vi "Measurement UI.vi"() -> ()   [LabVIEW 2021, in "Noise Sweep_Class D Amplifier_UI.lvlib"]
uses:
  Noise Sweep_Class D Amplifier_UI.lvlib
  shared/ui/controls/view.ctl
  shared/DAQmx/input terminal configuration.ctl
  UI State.ctl
  <vilib>/Utility/miscctls.llb/LVBoundsTypeDef.ctl
  <vilib>/Utility/miscctls.llb/LVPoint32TypeDef.ctl
  <vilib>/Utility/miscctls.llb/LVPointTypeDef.ctl
  shared/ui/UI Helpers.lvlib
  shared/audio popup ui/Audio Popup UI.lvlib
  shared/DAQmx/DAQmx utility.lvlib
panel:
  in  "view legend":T1
  out "plot point":string
  out "Sweep graph":cluster{"frequency (Hz)":dbl[], "THD+N":dbl[]}[](graph)
  out "Time domain graph":waveform(dbl)[](graph)
  out "channel names":string[](array[string])
  in  "digital serial cfg file":string
  in  "power supply resource":string="PXI1Slot4/ai0"
  out "idle channel noise (Vrms)":dbl[](array[numeric])
  out "power supply voltage (V)":dbl[](array[numeric])
  in  "Configuration tab":enum32{"Protocol", "Measurement"}(tab)
  out "digital serial file name":string
  in  "configure digital serial":bool
  in  "master clock channel list":string caption="Master Clock Channel"
  in  "digital channel list":string caption="Digital Audio Channel"
  in  "delay before measurement (s)":dbl=0.1 caption="Delay before measurement" format="%#_6ps"
  in  "input terminal cfg":T2 caption="Terminal Configuration"
  in  "input range":dbl=0.1 caption="Input range" format="%#_6g V"
  in  "power supply current limit":dbl caption="Current Limit" format="%#_g A"
  in  "power supply resource":refnum<k15> caption="Resource"
  in  "sweep number of steps":u32=20000 caption="Number of steps"
  in  "power supply voltage start":dbl=20.0 caption="Sweep start" format="%#_6p V"
  in  "power supply voltage stop":dbl=20000.0 caption="Sweep stop" format="%#_6g V"
  in  "Acquisition channel":tag
  in  "acq sampling rate":dbl=51200.0 caption="Sample rate" format="%#.6pHz"
  in  "measurement time (s)":dbl=0.1 caption="Minimum measurement time" format="%#_6ps"
  in  "weighting filter":T3(ring)=enum."A-weighting" caption="Weighting filter"
  out "wfm - data":dbl[](array[numeric])
  out "wfm - dt":dbl
  in  "acq channel":string="PXI1Slot4/ai0"
  # "hidden controls - used to sync with MeasLink"
  # "hidden indicators"
  # "Digital Serial Settings"
  # "Harware Resource"
  # "Power Supply Sweep"
  # "Filters"
  # "Acquisition"
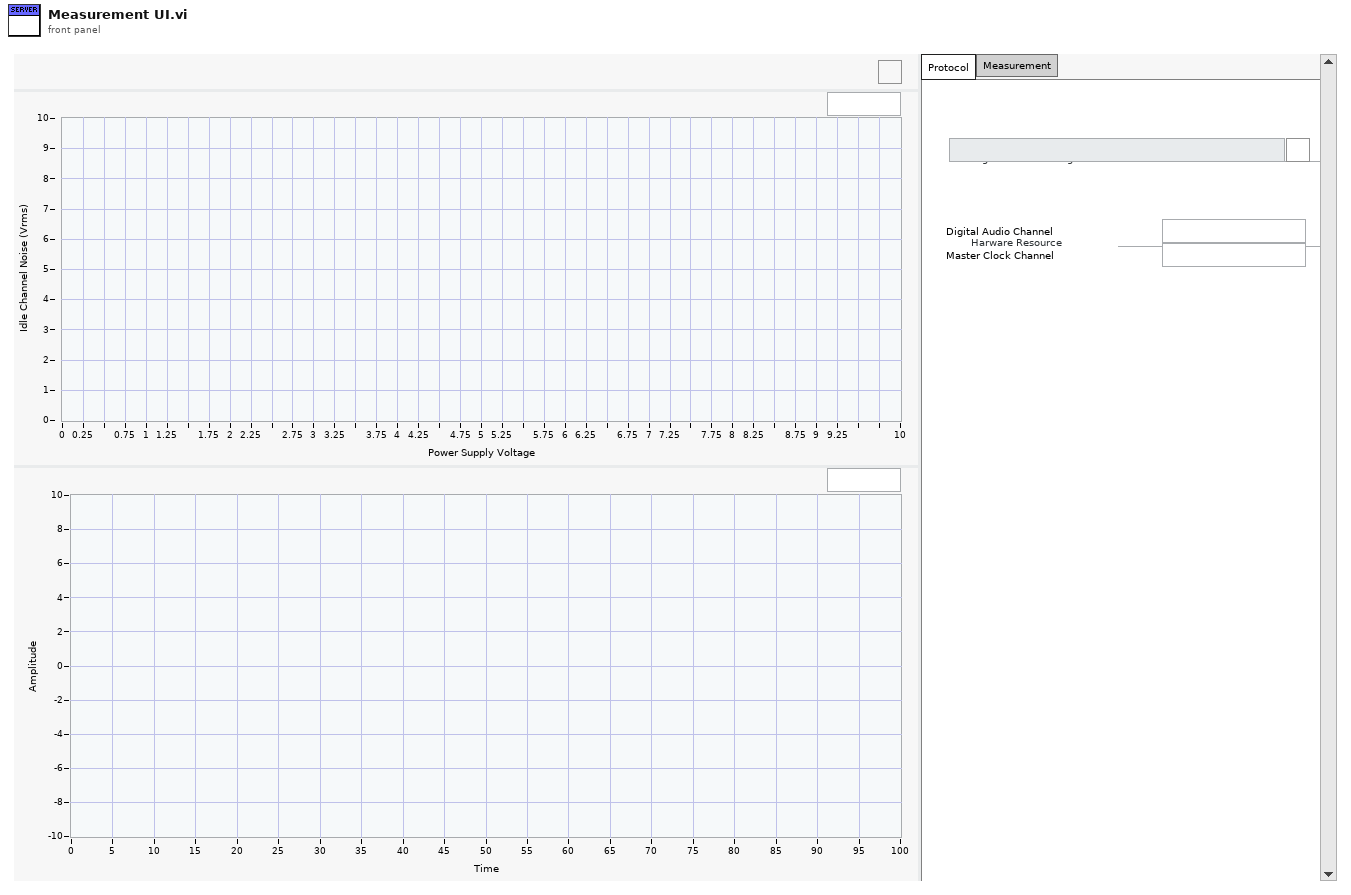
[diagram p1: front panel]
types:
  T1 = typedef "UI Helpers.lvlib/view.ctl" = bool
  T2 = typedef "DAQmx utility.lvlib/input terminal configuration.ctl" = enum32{"Default", "NRSE", "RSE", "Differential", "Pseudodifferential"}
  T3 = enum32{"Linear", "A-weighting", "B-weighting", "C-weighting"}
  T4 = typedef "Noise Sweep_Class D Amplifier_UI.lvlib/UI State.ctl" = cluster{"Graph Size":T5, "Legend Visible":bool, "Mouse Coords":T6, "Visible Plot Id":i32, "PostUI event occurred":bool, "digital serial cfg file":path}
  T5 = typedef "LVBoundsTypeDef.ctl" = cluster{"Width":u32, "Height":u32}
  T6 = typedef "LVPoint32TypeDef.ctl" = cluster{"Horizontal":i32, "Vertical":i32}
  T7 = typedef "LVPointTypeDef.ctl" = cluster{"Horizontal":i16, "Vertical":i16}
  T8 = typedef "Audio Popup UI.lvlib/audio settings.ctl" = cluster{"digital serial file":string}
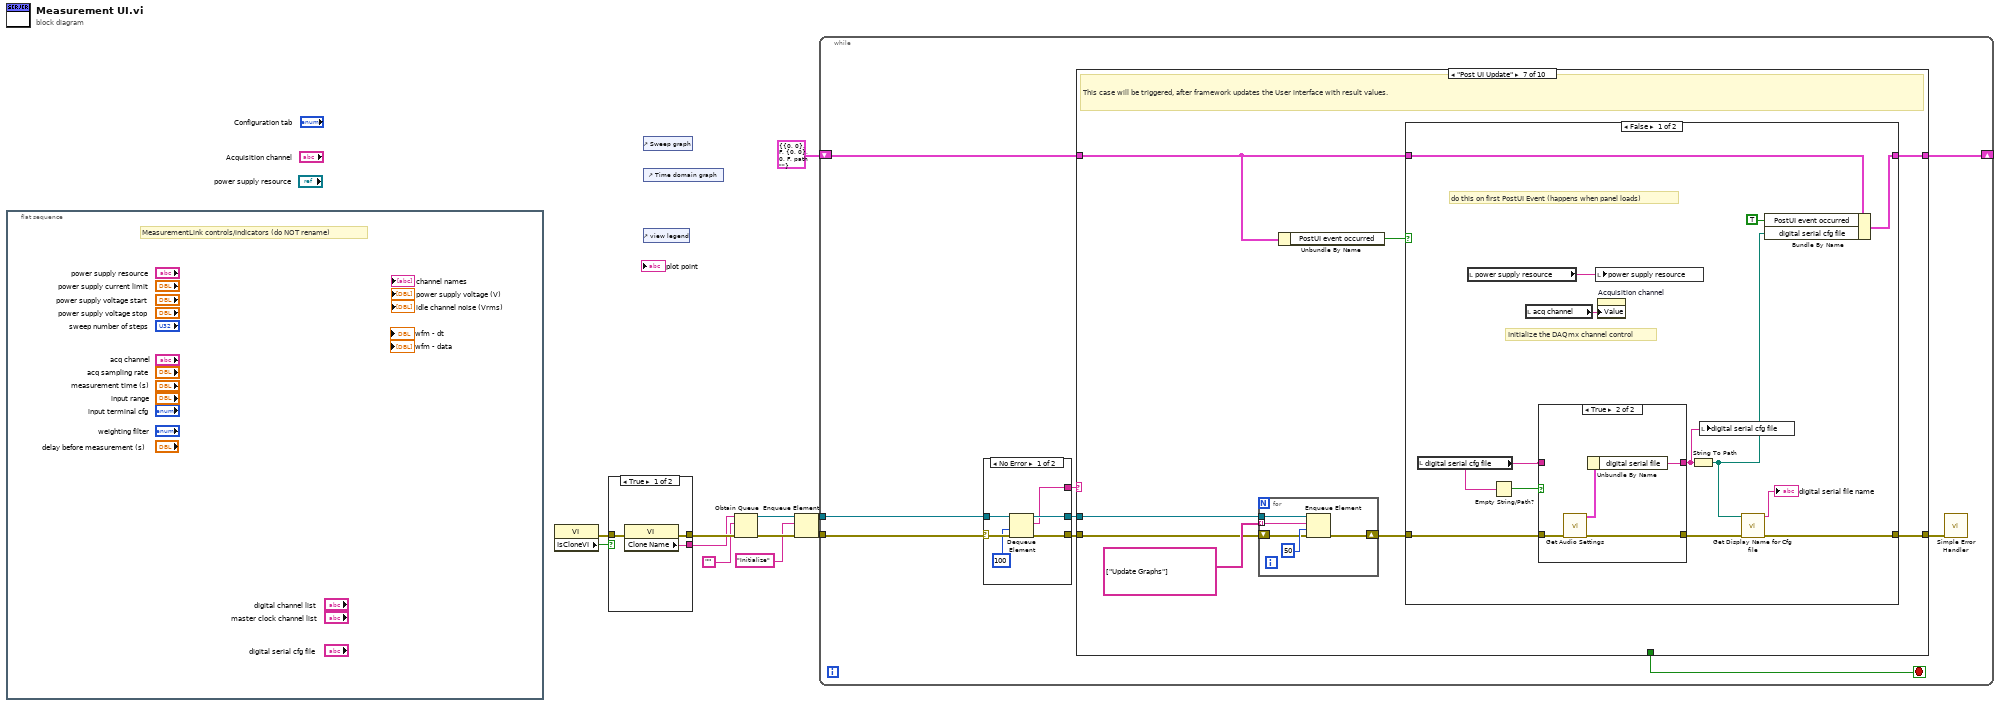
[diagram p0: block diagram]
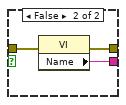
[diagram p2: hidden frame]
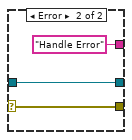
[diagram p3: hidden frame]
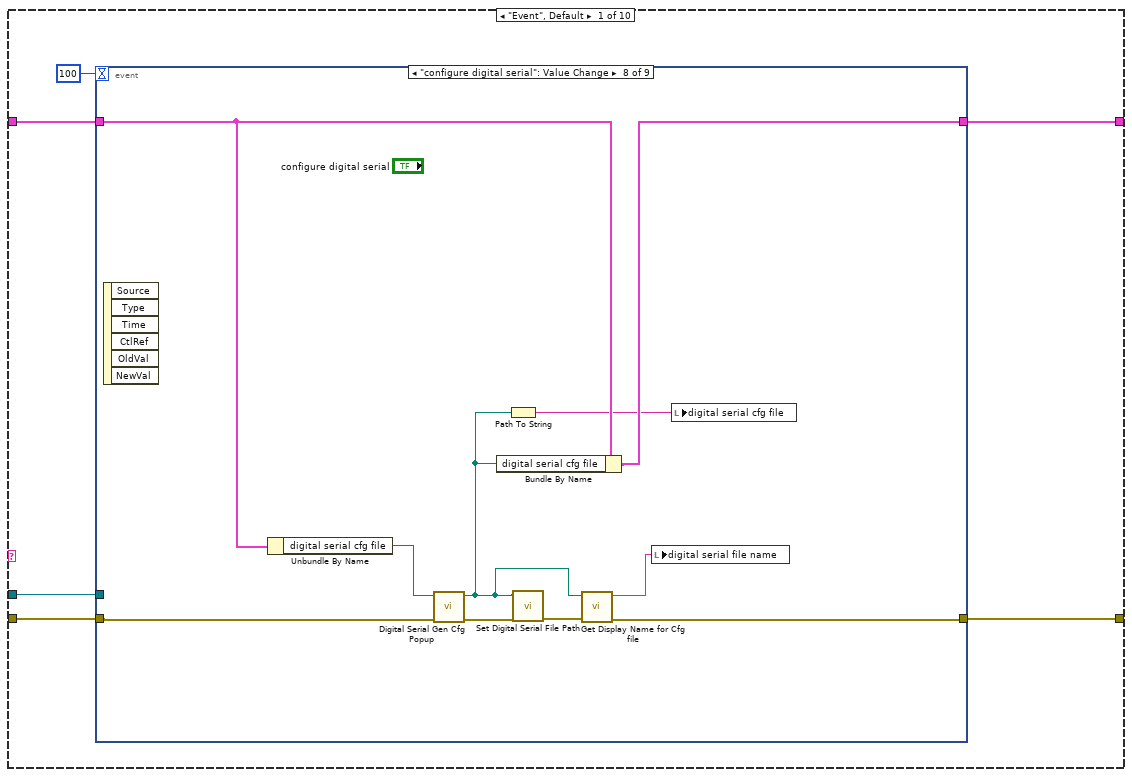
[diagram p4: hidden frame]
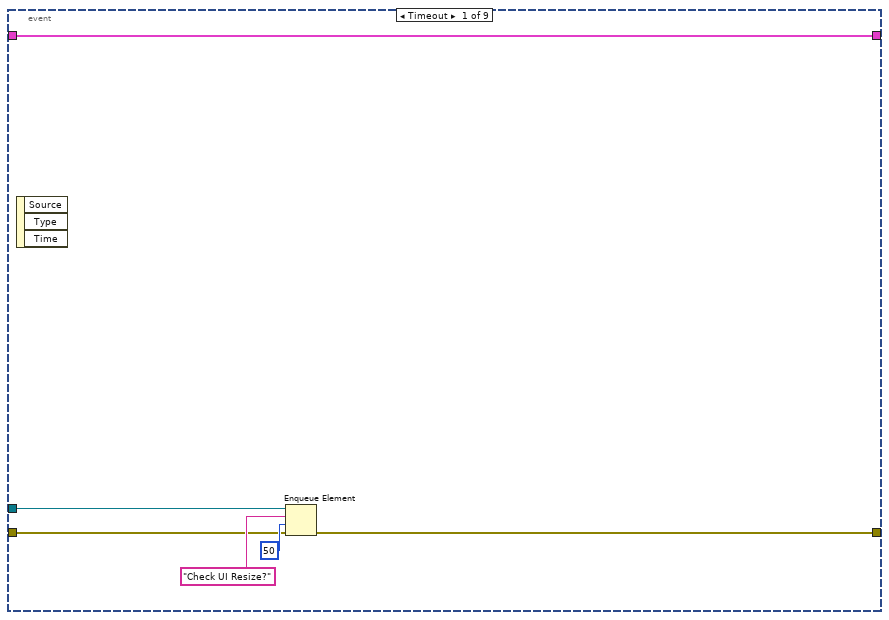
[diagram p5: hidden frame]
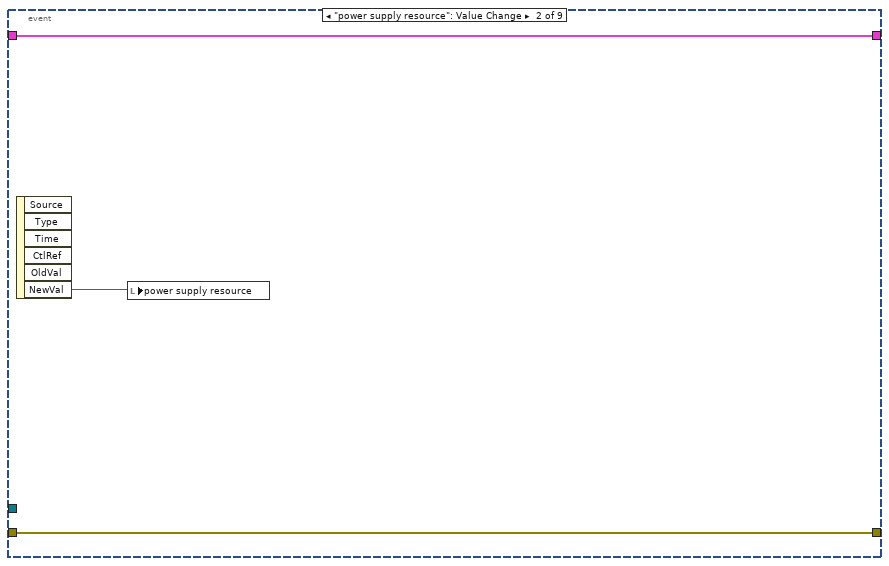
[diagram p6: hidden frame]
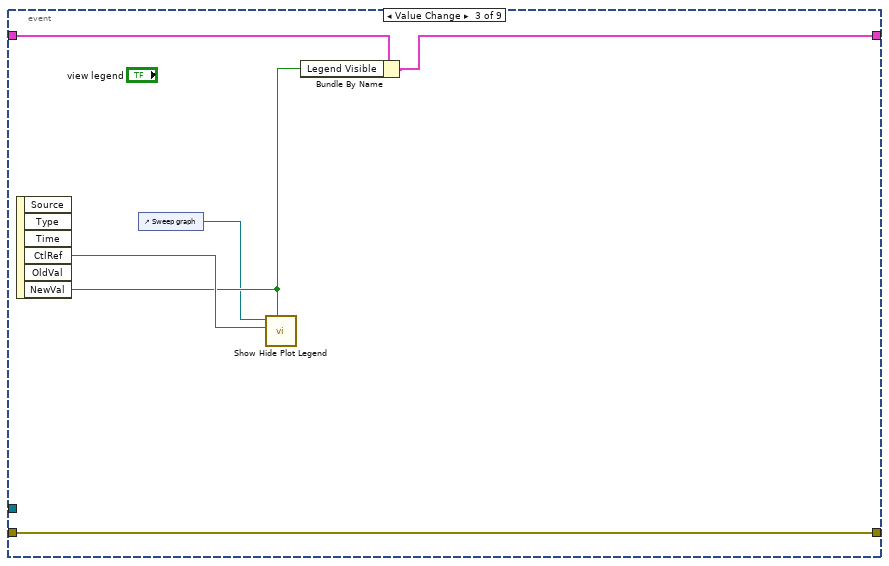
[diagram p7: hidden frame]
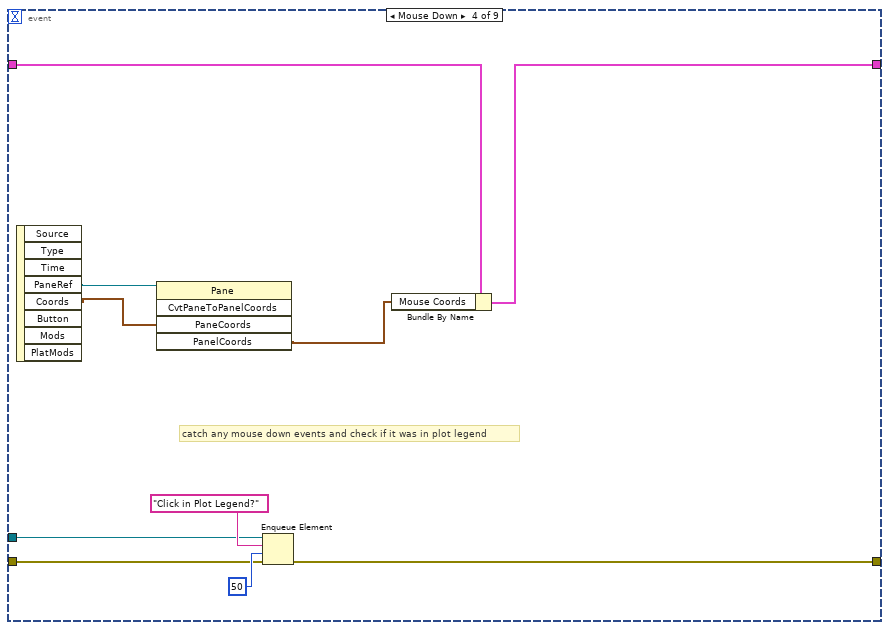
[diagram p8: hidden frame]
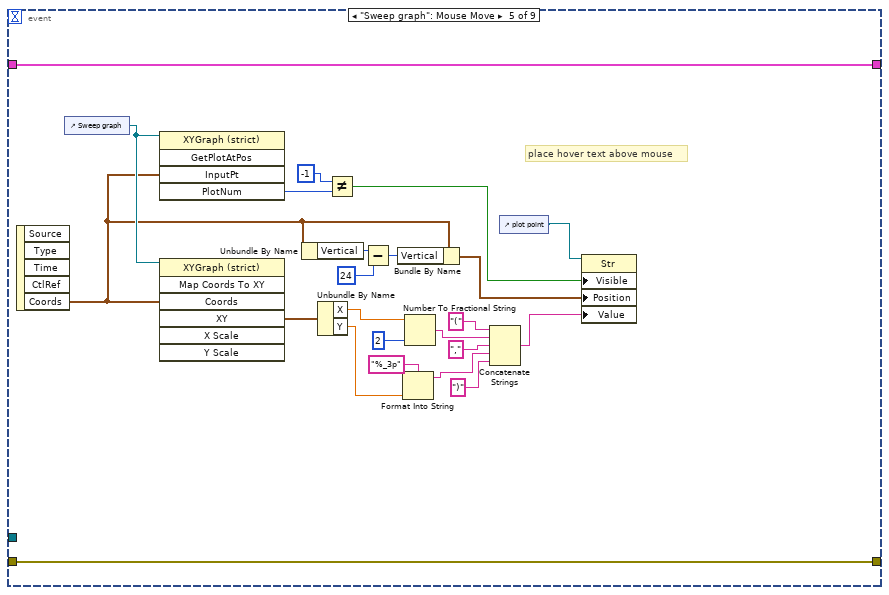
[diagram p9: hidden frame]
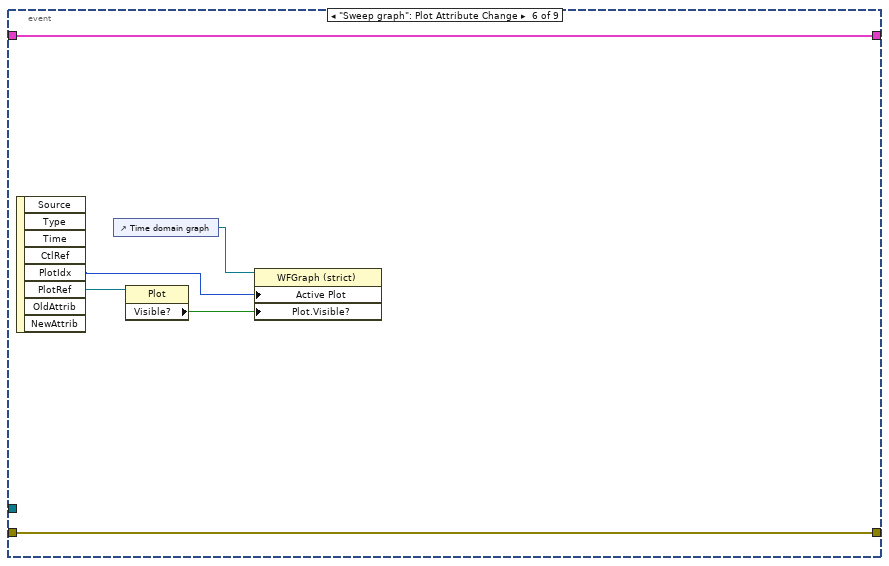
[diagram p10: hidden frame]
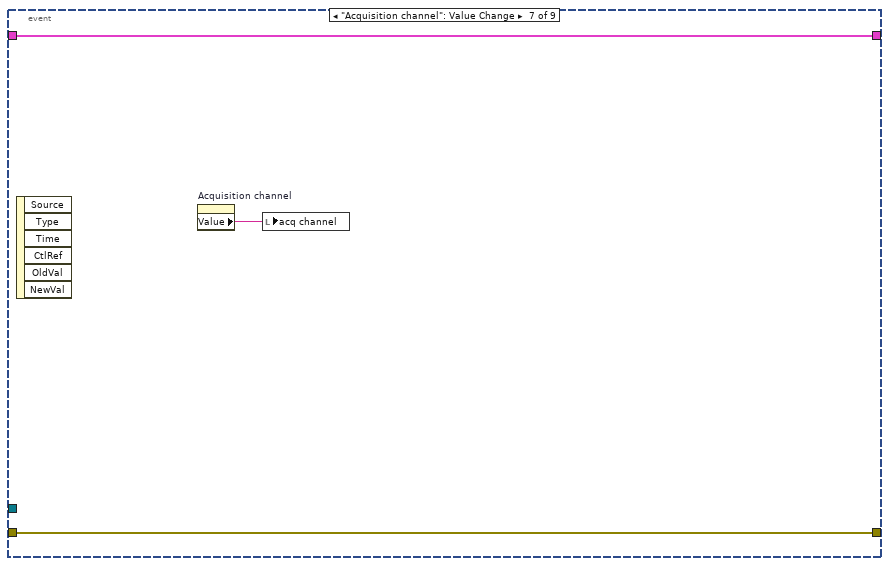
[diagram p11: hidden frame]
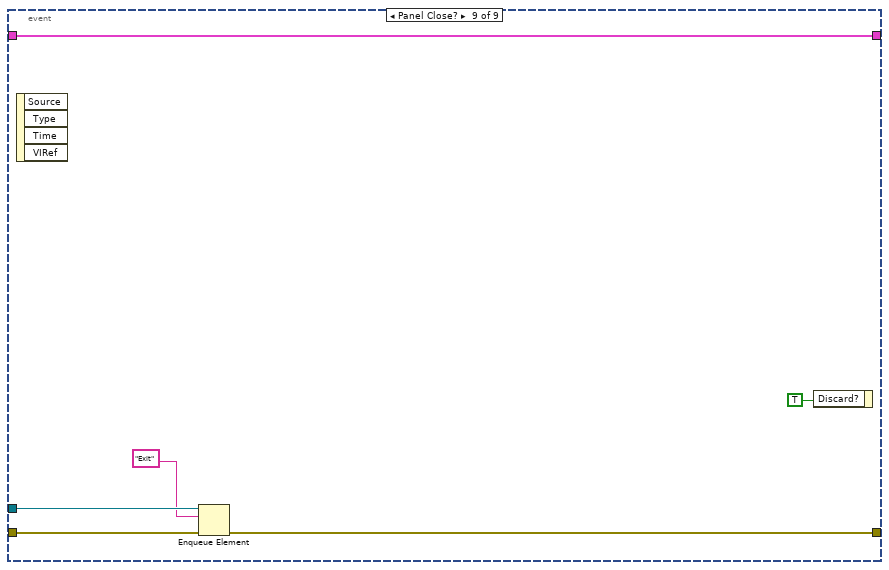
[diagram p12: hidden frame]
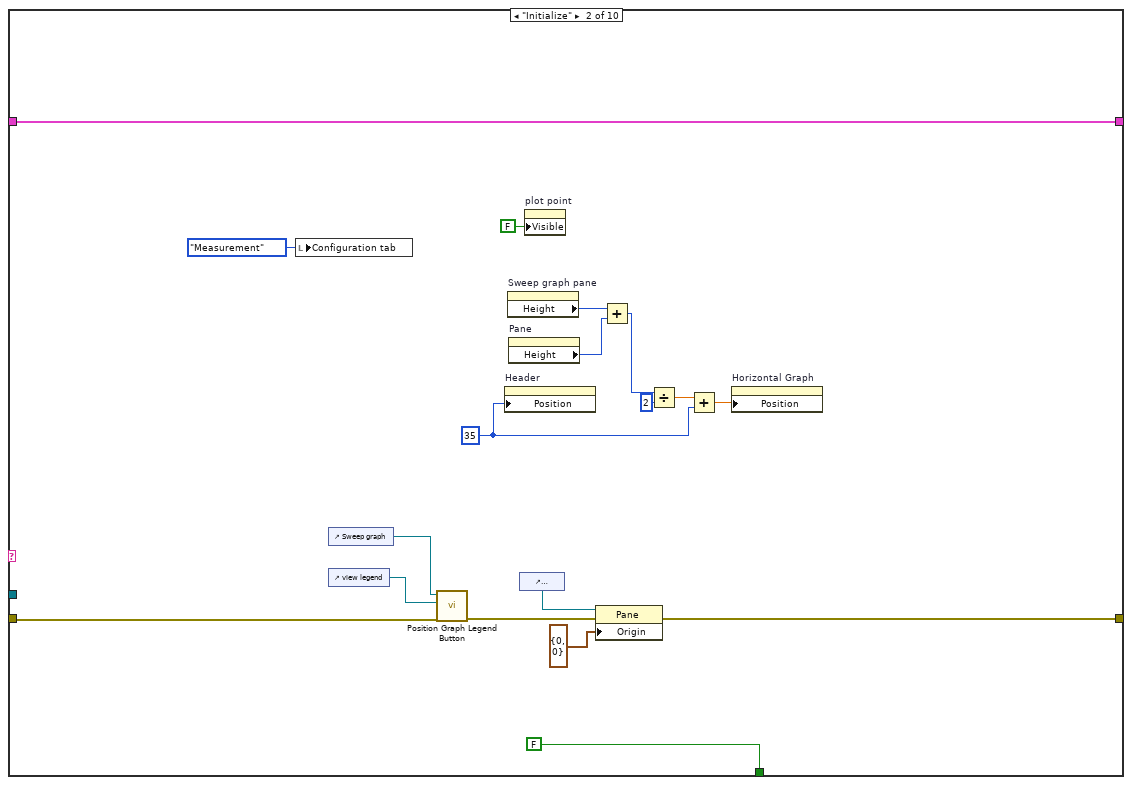
[diagram p13: hidden frame]
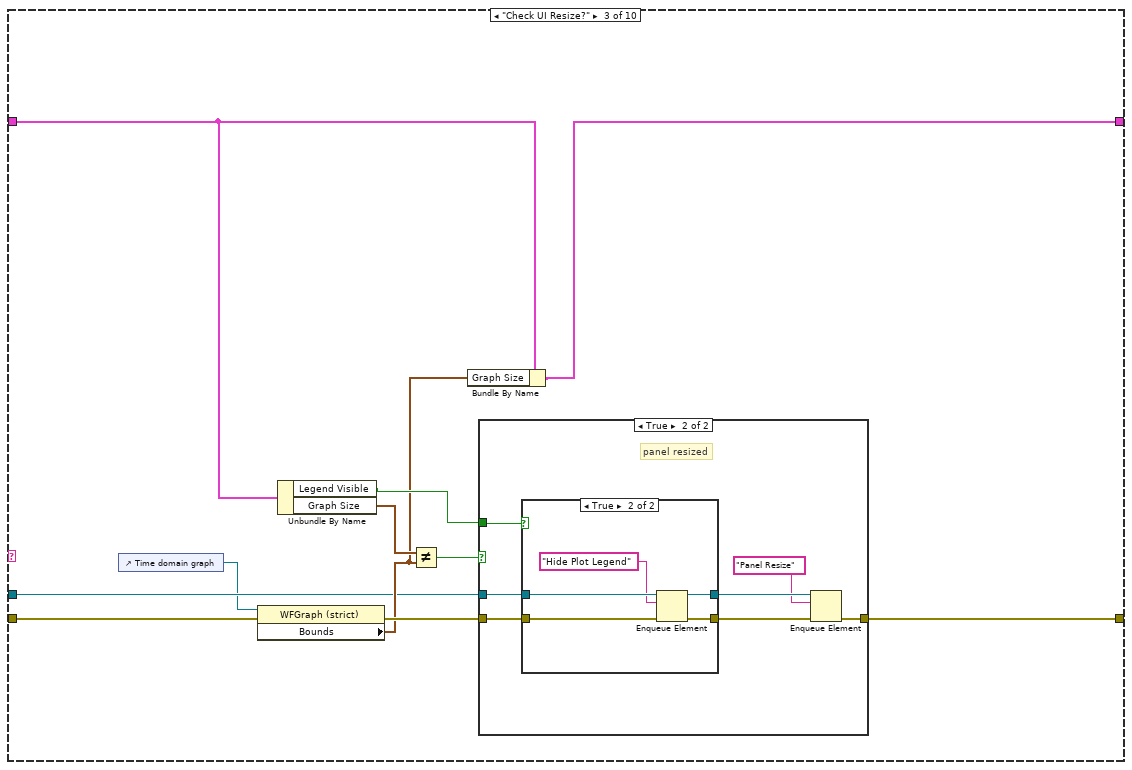
[diagram p14: hidden frame]
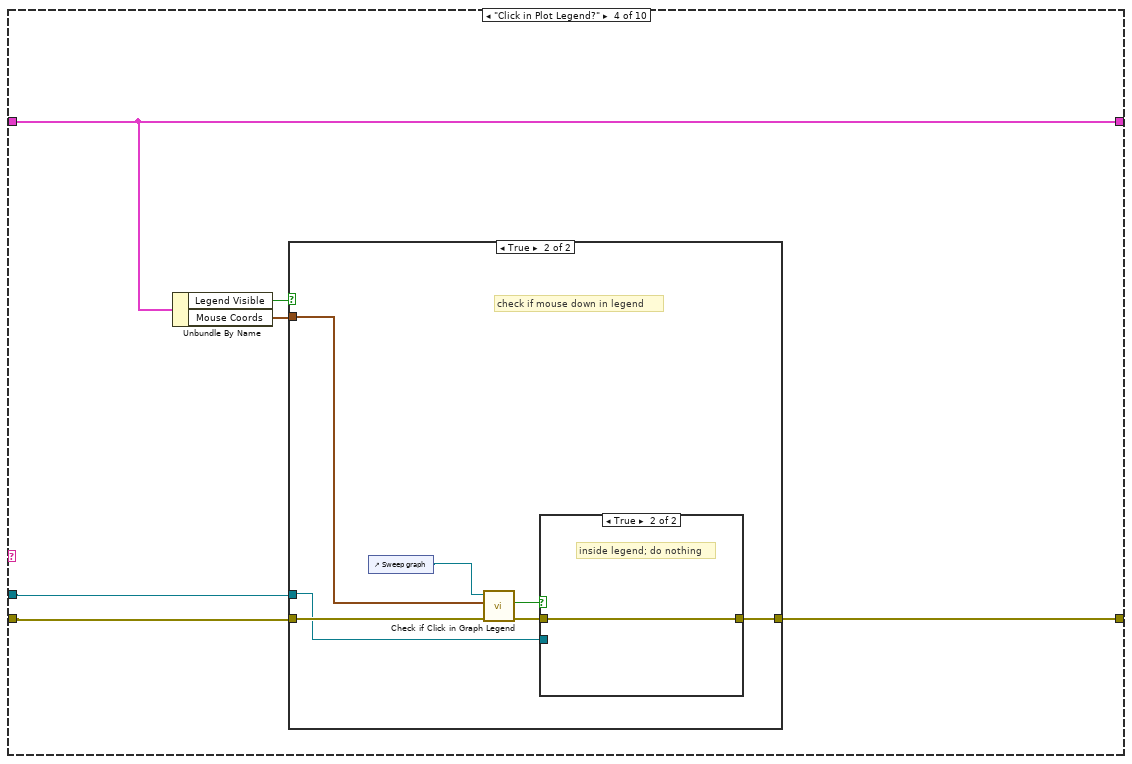
[diagram p17: hidden frame]
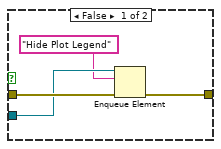
[diagram p19: hidden frame]
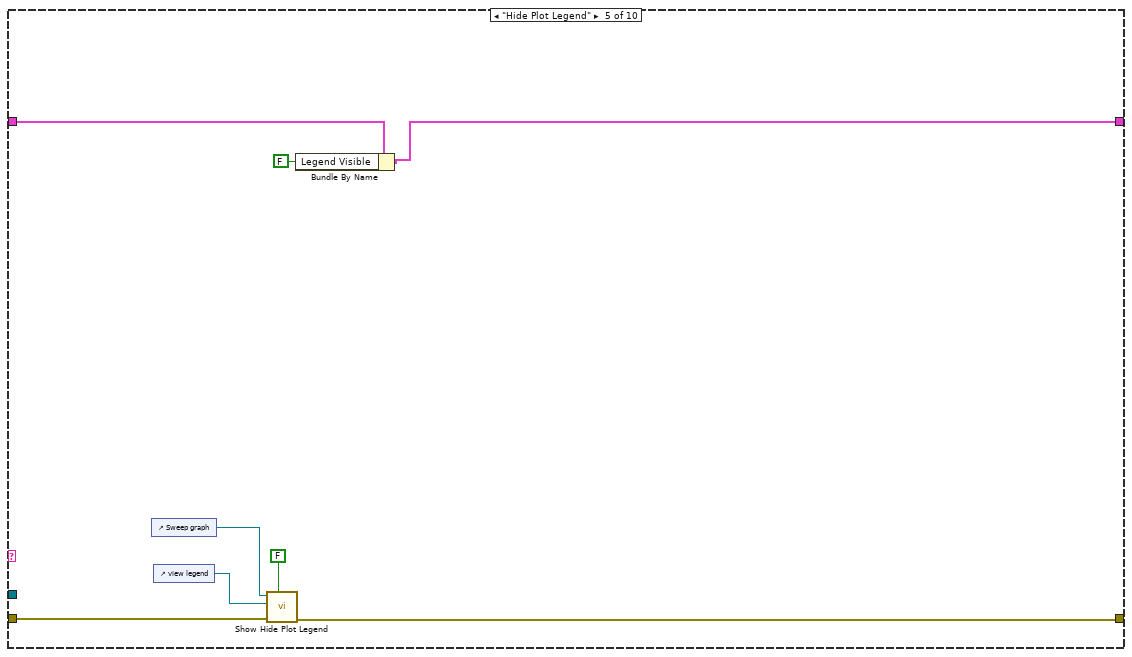
[diagram p20: hidden frame]
diagram:
  n1 = flat-sequence {
    frame #0 {
      # "MeasurementLink controls/indicators (do NOT rename)"
    }
  }
  n2 = property class="VI"() -> (error out=w2:errorcluster, "IsCloneVI"=w3:bool)  [unwired: 2 in, 1 out]
  n3 = case shown="True" w3 {
    tunnel: [w14 w17] -> w11
    tunnel: [w13 w16] -> w10
    tunnel: w2 -> [w12 w15]
    frame True {
      n4 = property class="VI"(error in=w12) -> (error out=w14:errorcluster, "Clone Name"=w13:string)  [unwired: 1 in, 1 out]
    }
    frame False {
      n5 = property class="VI"(error in=w15) -> (error out=w17:errorcluster, "Name"=w16:string)  [unwired: 1 in, 1 out]
    }
  }
  n6 = control-ref of="Sweep graph"() -> ()  [unwired: 1 out]
  n7 = control-ref of="Time domain graph"() -> ()  [unwired: 1 out]
  n8 = control-ref of="view legend"() -> ()  [unwired: 1 out]
  n9 = Obtain Queue(name (unnamed)=w10, element data type="", error in (no error)=w11) -> (queue out=w7:refnum<queue>, error out=w9:errorcluster)  [unwired: 2 in, 1 out]
  n10 = Enqueue Element(queue=w7, element="Initialize", error in (no error)=w9) -> (queue out=w6:refnum<queue>, error out=w8:errorcluster)  [unwired: 1 in, 1 out]
  n11 = while {
    tunnel: w6 -> [w24]
    shift-right: [w20] -> _
    shift-left: T4 {"Graph Size"={"Width"=0, "Height"=0}, "Legend Visible"=FALSE, "Mouse Coords"={"Horizontal"=0, "Vertical"=0}, "Visible Plot Id"=0, "PostUI event occurred"=FALSE, "digital serial cfg file"=path ""} ("UI State") -> [w19]
    tunnel: w8 -> [w26]
    stop <- w21 stop-if-true
    n12 = case shown="No Error" w26 {
      selector: w26 -> [w32 w35]
      tunnel: [w31 w35] -> w25
      tunnel: w24 -> [w30 w34]
      tunnel: [w29 w34] -> w23
      tunnel: [w28 "Handle Error"] -> w22
      frame No Error {
        n13 = Dequeue Element(queue=w30, timeout in ms (-1)=100, error in (no error)=w32) -> (queue out=w29:refnum<queue>, element=w28:string, error out=w31:errorcluster)  [unwired: 1 out]
      }
      frame Error {
      }
    }
    n14 = case shown="\"Post UI Update\"" w22 {
      tunnel: w25 -> [w40 w116 w137 w161 w181 w189 w197 w237 w253 w255]
      tunnel: w23 -> [w38 _ w138 w162 _ _ w196 _ w251 _]
      tunnel: [w41 w117 w136 w160 w180 w188 w191 w237 w248 w255] -> w18
      tunnel: [_ FALSE _ _ _ _ _ _ TRUE _] -> w21
      tunnel: [w36 w122 w133 w159 w183 w190 w194 w236 w246 w254] -> w20
      tunnel: w19 -> [w37 w122 w134 w159 w184 w190 w195 w236 w246 w254]
      frame "Event", Default {
        n15 = event shown="[7] \"configure digital serial\": Value Change" {
          selector: _ -> [_ _ _ _ _ _ _ _ _]
          dyn-events: _ -> [_ _ _ _ _ _ _ _ _]
          timeout: 100 -> [_ _ _ _ _ _ _ _ _]
          tunnel: [w44 w50 w56 w62 w89 w94 w96 w99 w112] -> w41
          tunnel: w40 -> [w45 w50 w56 w64 w89 w94 w96 w104 w113]
          tunnel: w38 -> [w43 _ _ w63 _ _ _ _ w111]
          tunnel: w37 -> [w42 w49 w53 w61 w88 w93 w97 w103 w109]
          tunnel: [w42 w49 w52 w60 w88 w93 w97 w102 w109] -> w36
          event Timeout {
            n16 = event-data() -> ()  [unwired: 1 in, 3 out]
            n17 = Enqueue Element(queue=w43, element="Check UI Resize?", timeout in ms (-1)=50, error in (no error)=w45) -> (error out=w44:errorcluster)  [unwired: 2 out]
          }
          event "power supply resource": Value Change {
            n18 = event-data() -> ("NewVal"=w48:refnum<k15>)  [unwired: 1 in, 5 out]
            n19 = local write "power supply resource"(w48) -> ()
          }
          event Value Change {
            n20 = event-data() -> ("CtlRef"=w55:refnum<vi>, "NewVal"=w54:T1)  [unwired: 1 in, 4 out]
            n21 = control-ref of="Sweep graph"() -> (w51:refnum<vi>)
            n22 = call "Show Hide Plot Legend.vi"("show"=w54, "view reference"=w55, "graph reference"=w51) -> ()  [unwired: 8 in, 1 out]
            n23 = Bundle By Name(cluster=w53, "Legend Visible"=w54) -> (w52:T4)
          }
          event Mouse Down {
            # "catch any mouse down events and check if it was in plot legend"
            n24 = event-data() -> ("PaneRef"=w59:refnum<vi>, "Coords"=w58:T6)  [unwired: 1 in, 6 out]
            n25 = invoke class="Pane" method="CvtPaneToPanelCoords"(reference=w59, "PaneCoords"=w58) -> ("PanelCoords"=w57:T7)  [unwired: 3 in, 4 out]
            n26 = Enqueue Element(queue=w63, element="Click in Plot Legend?", timeout in ms (-1)=50, error in (no error)=w64) -> (error out=w62:errorcluster)  [unwired: 2 out]
            n27 = Bundle By Name(cluster=w61, "Mouse Coords"=w57) -> (w60:T4)
          }
          event "Sweep graph": Mouse Move {
            # "place hover text above mouse"
            n28 = event-data() -> ("Coords"=w70:T6)  [unwired: 1 in, 4 out]
            n29 = control-ref of="Sweep graph"() -> (w71:refnum<vi>)
            n30 = invoke class="XYGraph (strict)" method="GetPlotAtPos"(reference=w71, "InputPt"=w70) -> ("PlotNum"=w86:i32)  [unwired: 3 in, 4 out]
            n31 = invoke class="XYGraph (strict)" method="Map Coords To XY"(reference=w71, "Coords"=w70) -> ("XY"=w87:cluster{"X":dbl, "Y":dbl})  [unwired: 5 in, 6 out]
            n32 = Unbundle By Name(w70) -> ("Vertical"=w75:i32)
            n33 = Unbundle By Name(w87) -> ("X"=w77:dbl, "Y"=w69:dbl)
            n34 = Not Equal?(x=-1, y=w86) -> (x != y?=w84:bool)
            n35 = Subtract(x=w75, y=24) -> (x-y=w74:i32)
            n36 = Bundle By Name(cluster=w70, "Vertical"=w74) -> (w76:T6)
            n37 = Format Into String(format string="%_3p", w69) -> (resulting string=w68:string)  [unwired: 2 in, 1 out]
            n38 = Number To Fractional String(number=w77, precision (6)=i16 2) -> (F-format string=w82:string)  [unwired: 2 in]
            n39 = Concatenate Strings("(" ("string"), w82, "," ("string"), w68, ")" ("string")) -> (w78:string)
            n40 = control-ref of="plot point"() -> (w72:refnum<vi>)
            n41 = property on="Property Node" class="Str"(reference=w72, "Visible"=w84, "Position"=w76, "Value"=w78) -> ()  [unwired: 1 in, 2 out]
          }
          event "Sweep graph": Plot Attribute Change {
            n42 = event-data() -> ("PlotIdx"=w92:i32, "PlotRef"=w95:refnum<vi>)  [unwired: 1 in, 6 out]
            n43 = control-ref of="Time domain graph"() -> (w90:refnum<vi>)
            n44 = property class="Plot"(reference=w95) -> ("Visible?"=w91:bool)  [unwired: 1 in, 2 out]
            n45 = property on="Property Node" class="WFGraph (strict)"(reference=w90, "Active Plot"=w92, "Plot.Visible?"=w91) -> ()  [unwired: 1 in, 2 out]
          }
          event "Acquisition channel": Value Change {
            n46 = event-data() -> ()  [unwired: 1 in, 6 out]
            n47 = property on="Acquisition channel" class="DAQmxName"() -> ("Value"=w98:string)  [unwired: 2 in, 2 out]
            n48 = local write "acq channel"(w98) -> ()
          }
          event "configure digital serial": Value Change {
            n49 = event-data() -> ()  [unwired: 1 in, 6 out]
            n50 = Unbundle By Name(w103) -> ("digital serial cfg file"=w108:path)
            n51 = call "Digital Serial Gen Cfg Popup.vi"("error in (no error)"=w104, "config file in"=w108) -> ("error out"=w107:errorcluster, "config file out"=w105:path)  [unwired: 7 in, 1 out]
            n52 = Bundle By Name(cluster=w103, "digital serial cfg file"=w105) -> (w102:T4)
            n53 = Path To String(path=w105) -> (string=w101:string)
            n54 = call "Set Digital Serial File Path.vi"("error in (no error)"=w107, "digital serial file"=w105) -> ("error out"=w106:errorcluster)  [unwired: 9 in]
            n55 = call "Get Display Name for Cfg file.vi"("error in (no error)"=w106, "file path"=w105) -> ("error out"=w99:errorcluster, "display string"=w100:string)  [unwired: 8 in]
            n56 = local write "digital serial file name"(w100) -> ()
            n57 = local write "digital serial cfg file"(w101) -> ()
          }
          event Panel Close? {
            n58 = event-data() -> ()  [unwired: 1 in, 4 out]
            n59 = Enqueue Element(queue=w111, element="Exit", error in (no error)=w113) -> (error out=w112:errorcluster)  [unwired: 1 in, 2 out]
            n60 = event-data("Discard?"=TRUE) -> ()  [unwired: 1 in, 1 out]
          }
        }
      }
      frame "Initialize" {
        w126 = 35 ("Splitter Position")
        n61 = local write "Configuration tab"(enum32{"Protocol", "Measurement"}."Measurement" ("Configuration tab")) -> ()
        n62 = control-ref of="Sweep graph"() -> (w127:refnum<vi>)
        n63 = control-ref of="view legend"() -> (w131:refnum<vi>)
        n64 = call "Position Graph Legend Button.vi"("error in (no error)"=w116, "view legend"=w131, "graph"=w127) -> ("error out"=w118:errorcluster)  [unwired: 8 in]
        n65 = property on="Header" class="Splitter"("Position"=w126) -> ()  [unwired: 2 in, 2 out]
        n66 = property on="Sweep graph pane" class="Pane"() -> ("Height"=w120:u32)  [unwired: 2 in, 2 out]
        n67 = property on="Pane" class="Pane"() -> ("Height"=w119:u32)  [unwired: 2 in, 2 out]
        n68 = control-ref of="Configuration Pane"() -> (w125:refnum<vi>)
        n69 = property on="plot point" class="Str"("Visible"=FALSE) -> ()  [unwired: 2 in, 2 out]
        n70 = property class="Pane"(reference=w125, error in=w118, "Origin"=T7 {"Horizontal"=0, "Vertical"=0}) -> (error out=w117:errorcluster)  [unwired: 1 out]
        n71 = Add(x=w120, y=w119) -> (x+y=w121:u32)
        n72 = Divide(x=w121, y=2) -> (x/y=w129:dbl)
        n73 = Add(x=w129, y=w126) -> (x+y=w128:dbl)
        n74 = property on="Horizontal Graph" class="Splitter"("Position"=w128) -> ()  [unwired: 2 in, 2 out]
      }
      frame "Check UI Resize?" {
        n75 = control-ref of="Time domain graph"() -> (w135:refnum<vi>)
        n76 = property on="Property Node" class="WFGraph (strict)"(reference=w135, error in=w137) -> (error out=w143:errorcluster, "Bounds"=w139:T5)  [unwired: 1 out]
        n77 = Unbundle By Name(w134) -> ("Legend Visible"=w141:bool, "Graph Size"=w140:T5)
        n78 = Not Equal?(x=w140, y=w139) -> (x != y?=w142:bool)
        n79 = Bundle By Name(cluster=w134, "Graph Size"=w139) -> (w133:T4)
        n80 = case shown="True" w142 {
          tunnel: w143 -> [w144 w151]
          tunnel: [w144 w146] -> w136
          tunnel: w141 -> [_ w149]
          tunnel: w138 -> [_ w150]
          frame False {
            # "no resize"
          }
          frame True {
            # "panel resized"
            n81 = case shown="True" w149 {
              tunnel: w151 -> [w153 w158]
              tunnel: [w153 w157] -> w148
              tunnel: w150 -> [w152 w156]
              tunnel: [w152 w154] -> w147
              frame False {
              }
              frame True {
                n82 = Enqueue Element(queue=w156, element="Hide Plot Legend", error in (no error)=w158) -> (queue out=w154:refnum<queue>, error out=w157:errorcluster)  [unwired: 1 in, 1 out]
              }
            }
            n83 = Enqueue Element(queue=w147, element="Panel Resize", error in (no error)=w148) -> (error out=w146:errorcluster)  [unwired: 1 in, 2 out]
          }
        }
      }
      frame "Click in Plot Legend?" {
        n84 = Unbundle By Name(w159) -> ("Legend Visible"=w163:bool, "Mouse Coords"=w164:T6)
        n85 = case shown="True" w163 {
          tunnel: w164 -> [_ w171]
          tunnel: w162 -> [_ w168]
          tunnel: w161 -> [w165 w172]
          tunnel: [w165 w167] -> w160
          frame False {
            # "legend not visible; do nothing"
          }
          frame True {
            # "check if mouse down in legend"
            n86 = control-ref of="Sweep graph"() -> (w166:refnum<vi>)
            n87 = call "Check if Click in Graph Legend.vi"("error in (no error)"=w172, "Mouse Coords"=w171, "WaveformGraph"=w166) -> ("error out"=w169:errorcluster, "click in legend?"=w170:bool)  [unwired: 7 in]
            n88 = case shown="True" w170 {
              tunnel: w169 -> [w176 w177]
              tunnel: w168 -> [w175 _]
              tunnel: [w174 w177] -> w167
              frame False {
                n89 = Enqueue Element(queue=w175, element="Hide Plot Legend", error in (no error)=w176) -> (error out=w174:errorcluster)  [unwired: 1 in, 2 out]
              }
              frame True {
                # "inside legend; do nothing"
              }
            }
          }
        }
      }
      frame "Hide Plot Legend" {
        n90 = control-ref of="Sweep graph"() -> (w178:refnum<vi>)
        n91 = control-ref of="view legend"() -> (w179:refnum<vi>)
        n92 = call "Show Hide Plot Legend.vi"("show"=FALSE, "error in (no error)"=w181, "view reference"=w179, "graph reference"=w178) -> ("error out"=w180:errorcluster)  [unwired: 7 in]
        n93 = Bundle By Name(cluster=w184, "Legend Visible"=FALSE ("legend visible")) -> (w183:T4)
      }
      frame "Panel Resize" {
        n94 = control-ref of="Sweep graph"() -> (w187:refnum<vi>)
        n95 = control-ref of="view legend"() -> (w186:refnum<vi>)
        n96 = call "Position Graph Legend Button.vi"("error in (no error)"=w189, "view legend"=w186, "graph"=w187) -> ("error out"=w188:errorcluster)  [unwired: 8 in]
      }
      frame "Post UI Update" {
        # "This case will be triggered, after framework updates the User interface with result values."
        n97 = for {
          tunnel: w196 -> [w222]
          shift-right: [w221] -> w192
          shift-left: w197 -> [w223]
          tunnel: string[] ["Update Graphs"] -> [w220] mode=indexing
          n98 = Enqueue Element(queue=w222, element=w220, timeout in ms (-1)=50, error in (no error)=w223) -> (error out=w221:errorcluster)  [unwired: 2 out]
        }
        n99 = Unbundle By Name(w195) -> ("PostUI event occurred"=w193:bool)
        n100 = case shown="False" w193 {
          tunnel: w195 -> [w211 w219]
          tunnel: [w210 w219] -> w194
          tunnel: w192 -> [w206 w218]
          tunnel: [w204 w218] -> w191
          frame False {
            # "Initialize the DAQmx channel control"
            # "do this on first PostUI Event (happens when panel loads)"
            n101 = local read "digital serial cfg file"() -> (w201:string)
            n102 = local read "power supply resource"() -> (w208:string)
            n103 = Empty String/Path?(string/path=w201) -> (empty?=w200:bool)
            n104 = local read "acq channel"() -> (w207:string)
            n105 = case shown="True" w200 {
              tunnel: w206 -> [w213 w217]
              tunnel: [w213 w215] -> w203
              tunnel: w201 -> [w212 _]
              tunnel: [w212 w214] -> w202
              frame False {
              }
              frame True {
                n106 = call "Get Audio Settings.vi"("error in (no error)"=w217) -> ("error out"=w215:errorcluster, "audio settings"=w216:T8)  [unwired: 9 in]
                n107 = Unbundle By Name(w216) -> ("digital serial file"=w214:string)
              }
            }
            n108 = local write "power supply resource"(w208) -> ()
            n109 = property on="Acquisition channel" class="DAQmxName"("Value"=w207) -> ()  [unwired: 2 in, 2 out]
            n110 = String To Path(string=w202) -> (path=w205:path)
            n111 = local write "digital serial cfg file"(w202) -> ()
            n112 = call "Get Display Name for Cfg file.vi"("error in (no error)"=w203, "file path"=w205) -> ("error out"=w204:errorcluster, "display string"=→"digital serial file name":string)  [unwired: 8 in]
            n113 = Bundle By Name(cluster=w211, "PostUI event occurred"=TRUE, "digital serial cfg file"=w205) -> (w210:T4)
          }
          frame True {
          }
        }
      }
      frame "Update Graphs" {
        n114 = local read "idle channel noise (Vrms)"() -> (w233:dbl[])
        n115 = local read "power supply voltage (V)"() -> (w234:dbl[])
        n116 = local read "channel names"() -> (w228:string[])
        n117 = local read "wfm - data"() -> (w232:dbl[])
        n118 = local read "wfm - dt"() -> (w231:dbl)
        n119 = control-ref of="Time domain graph"() -> (w229:refnum<vi>)
        n120 = call "Array to XY (N Ch).vi"("channel names"=w228, "Y data"=w233, "X data"=w234) -> ("XY plots"=→"Sweep graph":cluster{"X data":dbl[], "Y data":dbl[]}[])  [unwired: 8 in]
        n121 = call "Array to Wfm (N Ch).vi"("channel names"=w228, "dt"=w231, "array"=w232) -> ("waveforms"=→"Time domain graph":waveform(dbl)[])  [unwired: 8 in]
        n122 = Array Size(array=w228) -> (size(s)=w225:i32)
        n123 = for {
          tunnel: w229 -> [w243]
          tunnel: w228 -> [_] mode=indexing
          i -> [w244]
          # "make all plots visible"
          n124 = property class="WFGraph (strict)"(reference=w243, "Active Plot"=w244, "Plot.Visible?"=TRUE ("Plot.Visible")) -> ()  [unwired: 1 in, 2 out]
        }
        n125 = control-ref of="Sweep graph"() -> (w226:refnum<vi>)
        n126 = for {
          tunnel: w226 -> [w240]
          tunnel: w228 -> [w239] mode=indexing
          i -> [w242]
          n127 = property on="Property Node" class="XYGraph (strict)"(reference=w240, "Active Plot"=w242, "Plot.Plot Name"=w239, "Plot.Point Style"=u8 5, "Plot.Visible?"=TRUE ("Plot.Visible")) -> ()  [unwired: 1 in, 2 out]
        }
        n128 = property class="XYGraph (strict)"(reference=w226, "LegNumRows"=w225, "LegScrollVis"=FALSE ("Legend:Scrollbar Visible")) -> ()  [unwired: 1 in, 2 out]
      }
      frame "Exit" {
        # "This case is triggered to close the User Interface from framework"
        n129 = Flush Queue(queue=w251, error in (no error)=w253) -> (queue out=w250:refnum<queue>, error out=w249:errorcluster)  [unwired: 1 out]
        n130 = Release Queue(queue=w250, force destroy? (F)=TRUE, error in (no error)=w249) -> (error out=w248:errorcluster)  [unwired: 2 out]
      }
      frame "Handle Error" {
      }
    }
    n131 = call <vilib>:"Simple Error Handler.vi"("error in (no error)"=w18) -> ()  [unwired: 4 in, 5 out]
  }
